vi "Global Test.vi"() -> ()   [LabVIEW 2018, in "ICS.lvclass"]
uses:
  ICS.lvclass
panel:
  in  "End":u32=100
  in  "TX-RX":u32=100
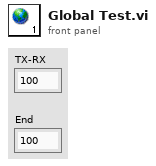
[diagram p1: front panel]
diagram:
